vi "HermiteGaussianBeam.vi"(0 "y_centre (in m; default 0)":dbl=0.000509999999999995 step=0.0001 format="%.5f", 2 "x_centre (in m; default 0)":dbl=0.0004899999999999976 step=0.0001 format="%.5f", 3 "beam waist w0 (in m; default 1E-4 = 0.1mm)":dbl=0.0001 format="%.2p", 4 "m":i16 min=0 step=1, 5 "n":i16 min=0 step=1, 6 "beam parameters":T1={"amplitudeMatrix"=[], "SLM width (m)"=0.01498, "SLM height (m)"=0.01092, "wavelength (m)"=6.33e-07, "Resolution x"=1920, "Resolution y"=1080} {"Resolution x" format="%#.0f"; "SLM width (m)" format="%_6f"; "SLM height (m)" format="%#_6f"}) -> (1 "Hermite-Gaussian beam":T1={"amplitudeMatrix"=[], "SLM width (m)"=0.01498, "SLM height (m)"=0.01092, "wavelength (m)"=6.33e-07, "Resolution x"=1920, "Resolution y"=1080} {"Resolution x" format="%#.0f"; "SLM width (m)" format="%_6f"; "SLM height (m)" format="%#_6f"})   [LabVIEW 2024]
uses:
  typeDefs/BPandSLM.ctl
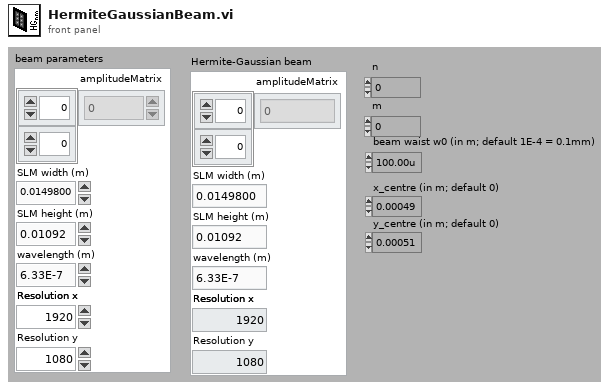
[diagram p1: front panel]
types:
  T1 = typedef "BPandSLM.ctl" = cluster{"amplitudeMatrix":csg[][], "SLM width (m)":dbl, "SLM height (m)":dbl, "wavelength (m)":dbl, "Resolution x":u32, "Resolution y":u32}
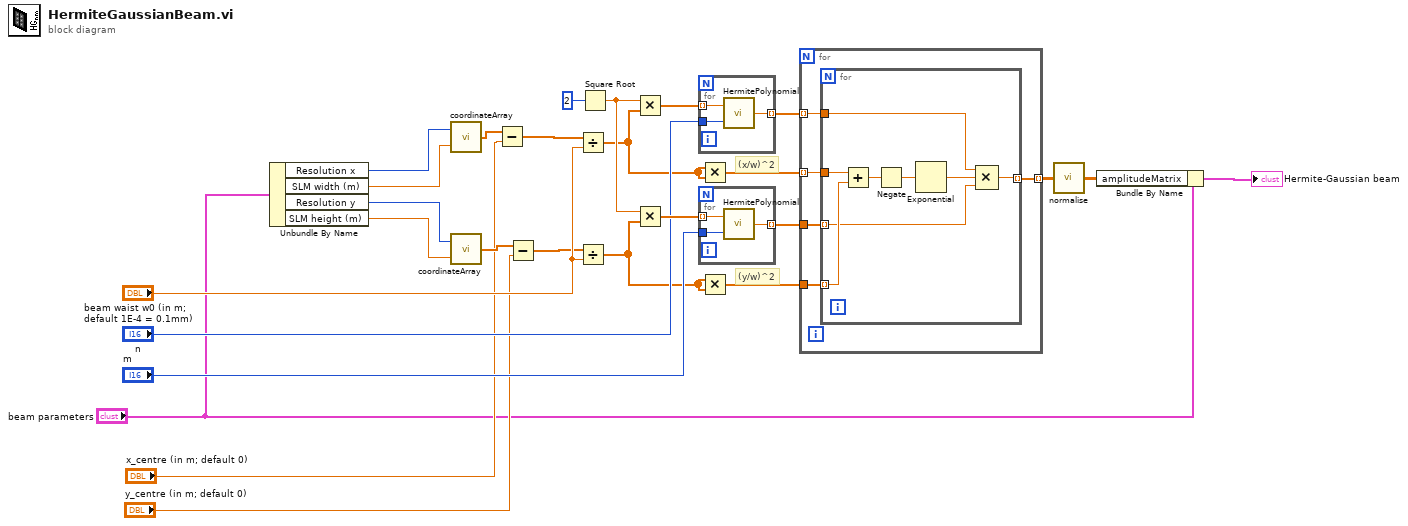
[diagram p0: block diagram]
diagram:
  # "(x/w)^2"
  # "(y/w)^2"
  n1 = Unbundle By Name("beam parameters") -> ("Resolution x"=w26:u32, "SLM width (m)"=w25:dbl, "Resolution y"=w24:u32, "SLM height (m)"=w23:dbl)
  n2 = call "coordinateArray.vi"("width of represented x (or y) range (in m; default 1E-3=1mm)"=w25, "array size (default 64)"=w26) -> ("x array"=w6:sgl[])
  n3 = call "coordinateArray.vi"("width of represented x (or y) range (in m; default 1E-3=1mm)"=w23, "array size (default 64)"=w24) -> ("x array"=w22:sgl[])
  n4 = Subtract(x=w6, y="x_centre (in m; default 0)") -> (x-y=w7:dbl[])
  n5 = Subtract(x=w22, y="y_centre (in m; default 0)") -> (x-y=w5:dbl[])
  n6 = Divide(x=w7, y="beam waist w0 (in m; default 1E-4 = 0.1mm)") -> (x/y=w11:dbl[])
  n7 = Divide(x=w5, y="beam waist w0 (in m; default 1E-4 = 0.1mm)") -> (x/y=w9:dbl[])
  n8 = Square Root(x=2) -> (sqrt(x)=w19:dbl)
  n9 = Multiply(x=w19, y=w11) -> (x*y=w16:dbl[])
  n10 = Multiply(x=w19, y=w9) -> (x*y=w18:dbl[])
  n11 = for {
    tunnel: w16 -> [w30] mode=indexing
    tunnel: "n" -> [w29]
    tunnel: [w28] -> w14 mode=indexing
    n12 = call "HermitePolynomial.vi"("n"=w29, "x"=w30) -> ("Hermite polynomial (n,x)"=w28:dbl)
  }
  n13 = for {
    tunnel: w18 -> [w33] mode=indexing
    tunnel: "m" -> [w32]
    tunnel: [w31] -> w13 mode=indexing
    n14 = call "HermitePolynomial.vi"("n"=w32, "x"=w33) -> ("Hermite polynomial (n,x)"=w31:dbl)
  }
  n15 = Multiply(x=w11, y=w11) -> (x*y=w12:dbl[])
  n16 = Multiply(x=w9, y=w9) -> (x*y=w10:dbl[])
  n17 = for {
    tunnel: w12 -> [w38] mode=indexing
    tunnel: w10 -> [w37]
    tunnel: [w36] -> w27 mode=indexing
    tunnel: w14 -> [w34] mode=indexing
    tunnel: w13 -> [w35]
    n18 = for {
      tunnel: w38 -> [w46]
      tunnel: w37 -> [w45] mode=indexing
      tunnel: [w40] -> w36 mode=indexing
      tunnel: w35 -> [w41] mode=indexing
      tunnel: w34 -> [w42]
      n19 = Add(x=w46, y=w45) -> (x+y=w44:dbl)
      n20 = Negate(x=w44) -> (-x=w43:dbl)
      n21 = Exponential(1:w43) -> (0:w39:dbl)
      n22 = Compound Arithmetic op=MULTIPLY(w42, w39, w41) -> (w40:dbl)
    }
  }
  n23 = call "normalise.vi"("amplitude matrix"=w27) -> ("normalised amplitude matrix"=w8:cdb[][])
  n24 = Bundle By Name(cluster="beam parameters", "amplitudeMatrix"=w8) -> (→"Hermite-Gaussian beam":T1)
